vi "Generate Trig pulse.vi"() -> ()   [LabVIEW 2020]
uses:
  <vilib>/rvi/eio/common/nirviEmuTemplateMethod_errors.vi
  <vilib>/rvi/Emulation/niFpgaGetClockAttributes.vi
  <vilib>/rvi/Emulation/niFpgaSctlEmulationGetInTimedLoop.vi
  <vilib>/rvi/Emulation/niFpgaEmulationReportErrorSimple.vi
  <vilib>/rvi/Emulation/niFpgaCriticalErrorInLSC.vi
  <vilib>/eio/EIONode/EIONode.xnode
panel:
  in  "stop":bool
  in  "TL Input":bool
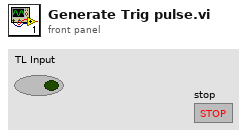
[diagram p1: front panel]
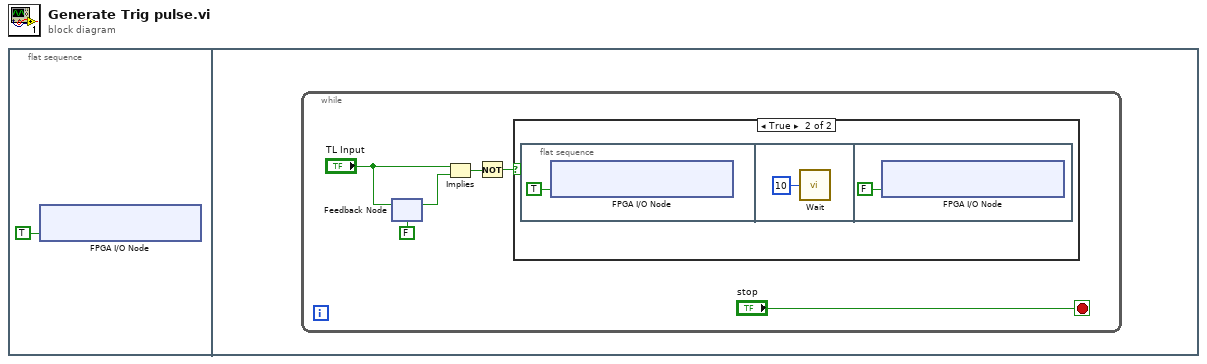
[diagram p0: block diagram]
diagram:
  n1 = flat-sequence {
    frame #0 {
      n2 = xnode "FPGA I/O Node"("IO Module\\Trigger WE"=TRUE ("IO Module\\Trigger WE")) -> ()  [unwired: 1 in, 1 out]
    }
    frame #1 {
      n3 = while {
        stop <- "stop" stop-if-true
        n4 = feedback #1(FALSE ("OK Button")) -> (w6:bool)
        n5 = feedback-in #1("TL Input") -> ()
        n6 = Implies(1:w6, 2:"TL Input") -> (0:w7:bool)
        n7 = Not(x=w7) -> (.not. x?=w3:bool)
        n8 = case shown="True" w3 {
          frame False {
          }
          frame True {
            n9 = flat-sequence {
              frame #0 {
                n10 = xnode "FPGA I/O Node"("IO Module\\Trigger Output"=TRUE ("IO Module\\Trigger Output")) -> ()  [unwired: 1 in, 1 out]
              }
              frame #1 {
                n11 = call "Wait"("Count(mSec)"=u32 10) -> ()  [unwired: 1 out]
              }
              frame #2 {
                n12 = xnode "FPGA I/O Node"("IO Module\\Trigger Output"=FALSE ("IO Module\\Trigger Output")) -> ()  [unwired: 1 in, 1 out]
              }
            }
          }
        }
      }
    }
  }
